vi "Is Created Queue.vi"(10 "Created Queue Alias":string, 11 "Base Event jettl in":refnum<class "Base Event jettl.lvclass">) -> (2 "Is Created Queue?":bool, 3 "Base Event jettl out":refnum<class "Base Event jettl.lvclass">)   [LabVIEW 2021, in "jettl.lvlib" / "Base Event jettl.lvlib" / "Base Event jettl.lvclass"]
uses:
  Base Event jettl.lvclass
  Base Event jettl.lvclass/Base Event jettl.ctl
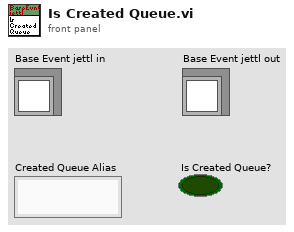
[diagram p1: front panel]
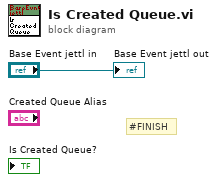
[diagram p0: block diagram]
diagram:
  # "#FINISH"
  "Base Event jettl out" <- "Base Event jettl in"
